vi "JSON Tree to ConnectionList.vi"(8 "error in (no error)":errorcluster, 11 "JSON Array":variant) -> (0 "error out":errorcluster, 2 "ConnectionList":T1[](array[typedef]), 3 "JSON Tree Passthrough (JSON Array)":variant)   [LabVIEW 2015, in "SLSC Switch.lvlib" / "SLSC Switch.lvclass"]
uses:
  SLSC Switch.lvclass
  Controls/JSON.ConnectionList.ctl
  <vilib>/LVH/i3 JSON/JSON Parsing/Get Object Parameter Files/Get Object Parameter - Array.vi
  <vilib>/LVH/i3 JSON/JSON Parsing/Get Array Value at Index Files/Get Array Value at Index - Object.vi
  <vilib>/LVH/i3 JSON/JSON Parsing/Get Object Parameter Files/Get Object Parameter - String.vi
  <vilib>/LVH/i3 JSON/i3-json.lvlib
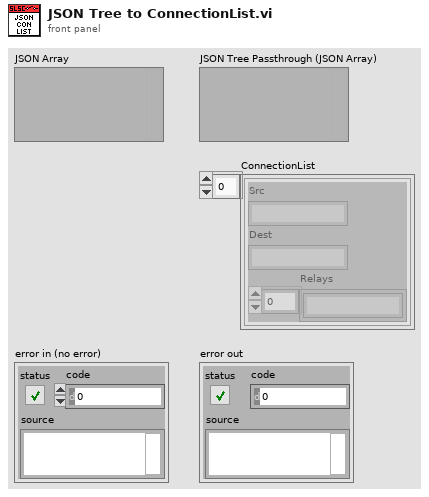
[diagram p1: front panel]
types:
  T1 = typedef "SLSC Switch.lvlib/SLSC Switch.lvclass/JSON.ConnectionList.ctl" = cluster{"Src":string, "Dest":string, "Relays":string[]}
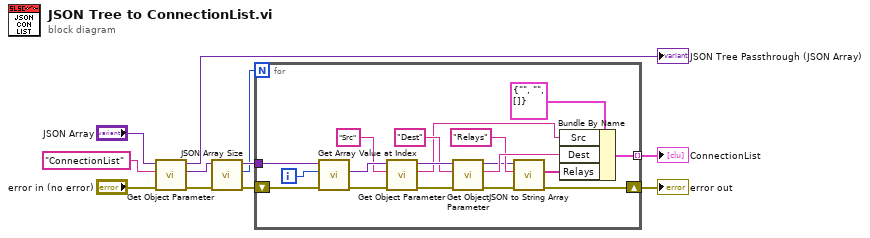
[diagram p0: block diagram]
diagram:
  n1 = call-poly <vilib>:"Get Object Parameter.vi"("error in (no error)"="error in (no error)", "Parameter Name"="ConnectionList", "JSON Tree In (JSON Object)"="JSON Array") -> ("error out"=w3:errorcluster, "JSON Array"=w2:variant, "JSON Tree Out Passthrough"=→"JSON Tree Passthrough (JSON Array)":variant)  [unwired: 5 in, 1 out]
  n2 = call <vilib>:"JSON Array Size.vi"("error in (no error)"=w3, "JSON Tree In (JSON Array)"=w2) -> ("error out"=w10:errorcluster, "Array Size"=w7:i32, "JSON Tree Passthrough (JSON Array)"=w8:variant)  [unwired: 7 in]
  n3 = for {
    N: w7 -> [_]
    tunnel: w8 -> [w29]
    tunnel: [w17] -> w9 mode=indexing
    shift-right: [w12] -> w11
    shift-left: w10 -> [w16]
    i -> [w28]
    n4 = call-poly <vilib>:"Get Array Value at Index.vi"("error in (no error)"=w16, "Index"=w28, "JSON Tree In (JSON Array)"=w29) -> ("error out"=w15:errorcluster, "JSON Object"=w27:variant)  [unwired: 5 in, 2 out]
    n5 = call-poly <vilib>:"Get Object Parameter.vi"("error in (no error)"=w15, "Parameter Name"="Src", "JSON Tree In (JSON Object)"=w27) -> ("error out"=w14:errorcluster, "String Value"=w22:string, "JSON Tree Out Passthrough"=w25:variant)  [unwired: 5 in, 1 out]
    n6 = call-poly <vilib>:"Get Object Parameter.vi"("error in (no error)"=w14, "Parameter Name"="Dest", "JSON Tree In (JSON Object)"=w25) -> ("error out"=w13:errorcluster, "String Value"=w21:string, "JSON Tree Out Passthrough"=w19:variant)  [unwired: 5 in, 1 out]
    n7 = call "JSON to String Array.vi"("error in (no error)"=w13, "Parameter Name"="Relays", "JSON Tree In"=w19) -> ("error out"=w12:errorcluster, "Array"=w18:string[])  [unwired: 6 in, 1 out]
    n8 = Bundle By Name(cluster=T1 {"Src"="", "Dest"="", "Relays"=[]} ("ConnectionList"), "Src"=w22, "Dest"=w21, "Relays"=w18) -> (w17:T1)
  }
  "error out" <- w11
  "ConnectionList" <- w9
